vi "Write TLS configuration.vi"(8 "error in (no error)":errorcluster, 10 "TLS configuration":refnum<k36>, 11 "TCPSocketBasedCommHandlerBase in":refnum<class "TCPSocketBasedCommHandlerBase.lvclass">) -> (0 "error out":errorcluster, 3 "TCPSocketBasedCommHandlerBase out":refnum<class "TCPSocketBasedCommHandlerBase.lvclass">)   [LabVIEW 2020]
uses:
  TCPSocketBasedCommHandlerBase.lvclass
  TCPSocketBasedCommHandlerBase.lvclass/TCPSocketBasedCommHandlerBase.ctl
  C:/local/wamplv/Private/Comm Handlers/CommHandlerBase/CommHandlerBase.lvclass
  C:/local/wamplv/Private/Comm Handlers/ICommHandler/ICommHandler.lvclass
  C:/local/wamplv/Private/Comm Handlers/TCPSocketBasedCommHandlerBase/TCPSocketBasedCommHandlerBase.lvclass
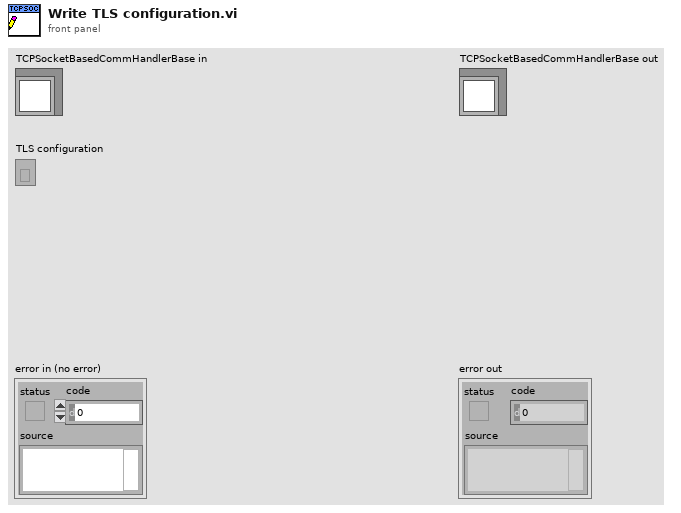
[diagram p1: front panel]
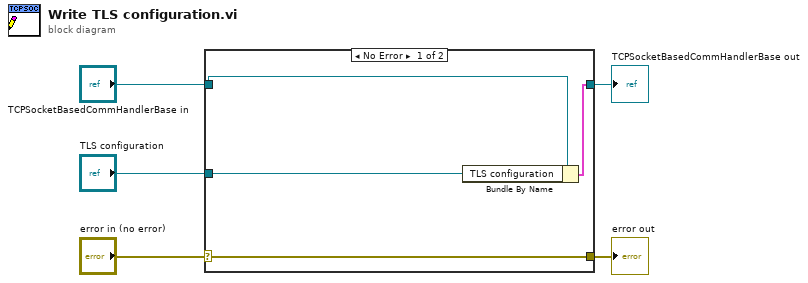
[diagram p0: block diagram]
diagram:
  n1 = case shown="No Error" "error in (no error)" {
    selector: "error in (no error)" -> [w9 w10]
    tunnel: [w9 w10] -> w4
    tunnel: [w7 w11] -> w2
    tunnel: "TCPSocketBasedCommHandlerBase in" -> [w8 w11]
    tunnel: "TLS configuration" -> [w6 _]
    frame No Error {
      n2 = Bundle By Name(cluster=w8, "TLS configuration"=w6) -> (w7:cluster{})
    }
    frame Error {
    }
  }
  "error out" <- w4
  "TCPSocketBasedCommHandlerBase out" <- w2
